vi "Write Position.vi"(8 "error in (no error)":errorcluster, 10 "Position":cluster{"Left":i32, "Top":i32}, 11 "Layered Shape in":refnum<class "Layered Shape.lvclass">) -> (0 "error out":errorcluster, 3 "Layered Shape out":refnum<class "Layered Shape.lvclass">)   [LabVIEW 2017, in "LV Image Editor Framework.lvlib" / "Layered Shape.lvclass"]
uses:
  Layered Shape.lvclass
  Layered Shape.lvclass/Layered Shape.ctl
  Shape/Shape.lvclass
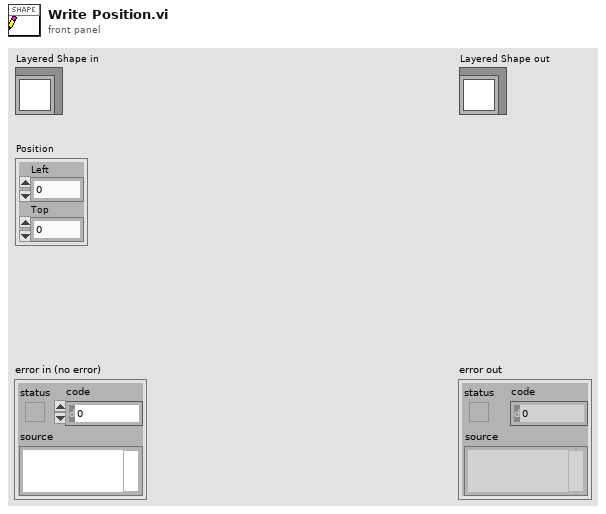
[diagram p1: front panel]
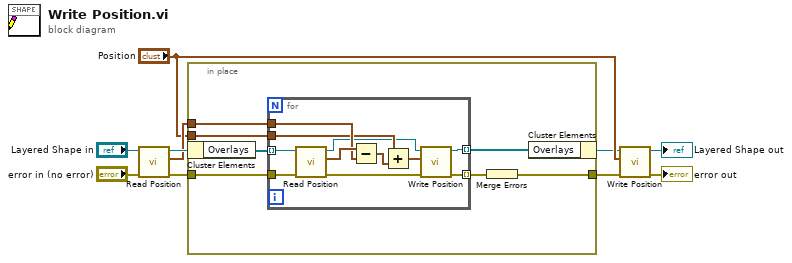
[diagram p0: block diagram]
diagram:
  n1 = call-dynamic "Read Position.vi"("error in (no error)"="error in (no error)", "Shape in"="Layered Shape in") -> ("error out"=w4:errorcluster, "Position"=w6:cluster{"Left":i32, "Top":i32}, "Shape out"=w7:refnum<class "Layered Shape.lvclass">)  [unwired: 7 in]
  n2 = in-place {
    in-place-border: w6 -> [w16]
    in-place-border: "Position" -> [w15]
    in-place-border: w4 -> [w14]
    in-place-border: [w11] -> w2
    n3 = in-place-cluster #1(w7) -> ("Overlays"=w17:refnum<class "Shape.lvclass">[])
    n4 = for {
      tunnel: w17 -> [w28] mode=indexing
      tunnel: w16 -> [w26]
      tunnel: w15 -> [w24]
      tunnel: w14 -> [w21]
      tunnel: [w20] -> w13 mode=indexing
      tunnel: [w19] -> w12 mode=indexing
      n5 = call-dynamic "Read Position.vi"("error in (no error)"=w21, "Shape in"=w28) -> ("error out"=w22:errorcluster, "Position"=w27:cluster{"Left":i32, "Top":i32}, "Shape out"=w23:refnum<class "Shape.lvclass">)  [unwired: 7 in]
      n6 = Subtract(x=w27, y=w26) -> (x-y=w25:cluster{"Left":i32, "Top":i32})
      n7 = Add(x=w24, y=w25) -> (x+y=w18:cluster{"Left":i32, "Top":i32})
      n8 = call-dynamic "Write Position.vi"("error in (no error)"=w22, "Position"=w18, "Shape in"=w23) -> ("error out"=w19:errorcluster, "Shape out"=w20:refnum<class "Shape.lvclass">)  [unwired: 7 in]
    }
    n9 = Merge Errors(w12) -> (w11:errorcluster)
    n10 = in-place-cluster #1("Overlays"=w13) -> (w1:refnum<class "Layered Shape.lvclass">)
  }
  n11 = call-parent "Write Position.vi"("error in (no error)"=w2, "Position"="Position", "Shape in"=w1) -> ("error out"=→"error out":errorcluster, "Shape out"=→"Layered Shape out":refnum<class "Layered Shape.lvclass">)  [unwired: 7 in]
